vi "Read Autoscale Delay.vi"(9 "GraphChart in":refnum<class "GraphChart.lvclass">) -> (3 "GraphChart out":refnum<class "GraphChart.lvclass">, 4 "Autoscale Delay":sgl)   [LabVIEW 2014, in "Raspberry Pi Compatible Compiler for LabVIEW.lvlib" / "GraphChart.lvclass"]
uses:
  GraphChart.lvclass
  GraphChart.lvclass/GraphChart.ctl
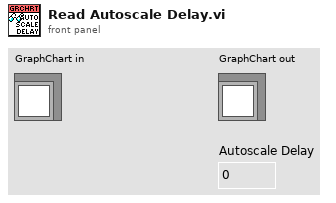
[diagram p1: front panel]
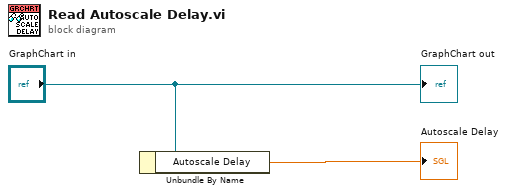
[diagram p0: block diagram]
diagram:
  n1 = Unbundle By Name("GraphChart in") -> ("Autoscale Delay"=→"Autoscale Delay":sgl)
  "GraphChart out" <- "GraphChart in"
